vi "load vi modification tools.vi"() -> ()   [LabVIEW 2013, in "vi mod UI.lvlib"]
uses:
  vi mod UI.lvlib
  VI modification.lvclass
panel:
  in  "Remove path":bool
  in  "add search":bool
  in  "Paths":i32(listbox)
  in  "run":bool
  in  "remove":bool
  in  "add":bool
  in  "Selected Tools":i32(listbox)
  in  "Available Tools":i32(listbox)
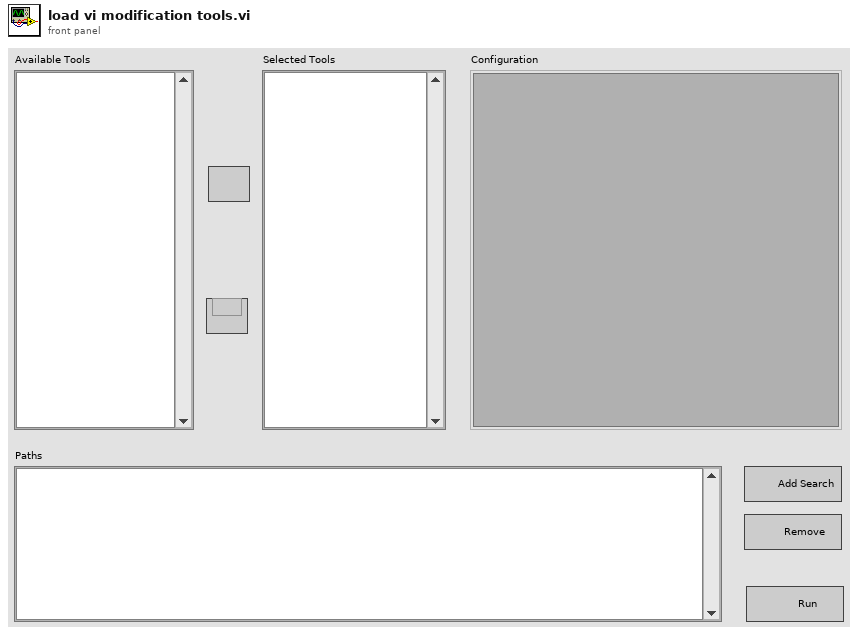
[diagram p1: front panel]
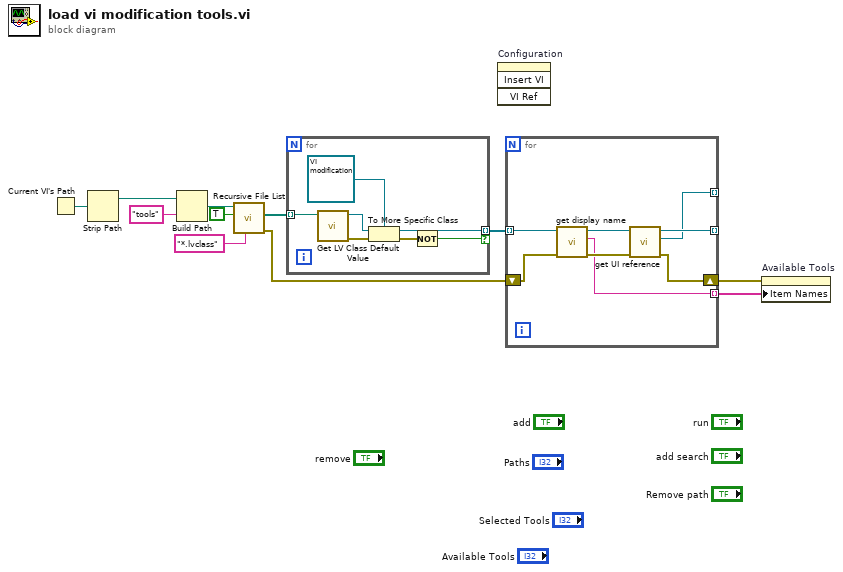
[diagram p0: block diagram]
diagram:
  n1 = Current VI's Path() -> (path=w11:path)
  n2 = Strip Path(path=w11) -> (stripped path=w10:path)  [unwired: 1 out]
  n3 = Build Path(base path=w10, name or relative path="tools") -> (appended path=w8:path)
  n4 = call <vilib>:"Recursive File List.vi"("pattern"="*.lvclass", "Treat LLBs as Folders?"=TRUE, "Folder Path"=w8) -> ("error out"=w3:errorcluster, "All Files in Dir"=w5:path[])  [unwired: 4 in, 3 out]
  n5 = for {
    tunnel: w5 -> [w18] mode=indexing
    tunnel: [w14] -> w4 mode=indexing if=w12
    n6 = call <vilib>:"Get LV Class Default Value.vi"("class path"=w18) -> ("error out"=w17:errorcluster, "object"=w16:refnum<class>)  [unwired: 9 in]
    n7 = To More Specific Class(target class=refnum<class "VI modification.lvclass"> refnum ("VI modification"), reference=w16, error in=w17) -> (specific class reference=w14:refnum<class "VI modification.lvclass">, error out=w13:errorcluster)
    n8 = Not(x=w13) -> (.not. x?=w12:bool)
  }
  n9 = invoke on="Configuration" class="SubPanel" method="Insert VI"() -> ()  [unwired: 4 in, 4 out]
  n10 = for {
    tunnel: w4 -> [w26] mode=indexing
    shift-right: [w23] -> w2
    shift-left: w3 -> [w25]
    tunnel: [w21] -> _ mode=indexing
    tunnel: [w20] -> w1 mode=indexing
    tunnel: [w19] -> _ mode=indexing
    n11 = call-dynamic "get display name.vi"("error in"=w25, "VI modification in"=w26) -> ("error out"=w24:errorcluster, "class name"=w20:string, "VI modification out"=w22:refnum<class "VI modification.lvclass">)  [unwired: 7 in]
    n12 = call-dynamic "get UI reference.vi"("error in"=w24, "VI modification in"=w22) -> ("error out"=w23:errorcluster, "VI Refnum"=w19:refnum<vi>, "VI modification out"=w21:refnum<class "VI modification.lvclass">)  [unwired: 7 in]
  }
  n13 = property on="Available Tools" class="LstBox (strict)"(error in=w2, "Item Names"=w1) -> ()  [unwired: 1 in, 2 out]
